vi "ReversePoly.vi"   [LabVIEW 2022 SP3]
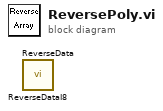
[diagram p0: block diagram]
diagram:
  n1 = call "ReverseDataI8.vi"() -> ()  [unwired: 1 in, 1 out]
  n2 = call "ReverseData.vi"() -> ()  [unwired: 1 in, 1 out]
